vi "C8855-01_InitCall.vi"() -> (0 "ExtT":bool, 1 "Moni":bool, 2 "Measur":u32, 3 "GT":i32, 4 "TrgEdge":u8)   [LabVIEW 2017]
panel:
  out "InitFN":string
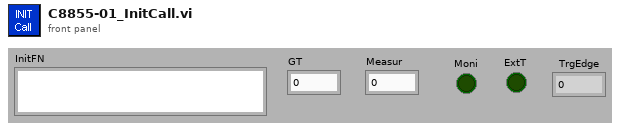
[diagram p1: front panel]
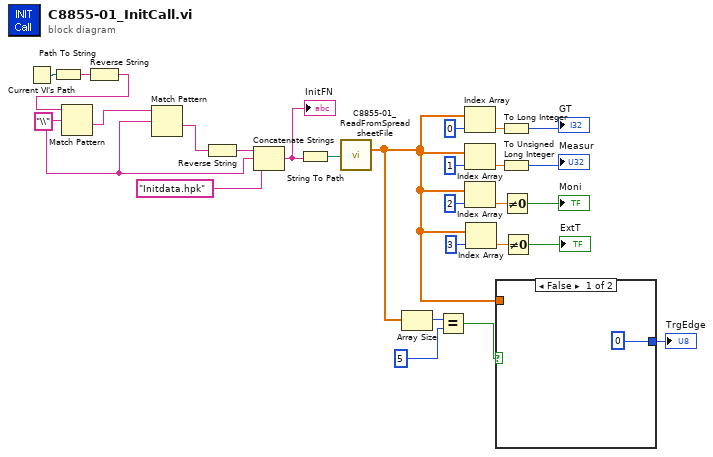
[diagram p0: block diagram]
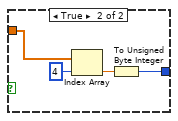
[diagram p2: hidden frame]
diagram:
  w20 = "\\" ("regular expression")
  n1 = Current VI's Path() -> (path=w27:path)
  n2 = Path To String(path=w27) -> (string=w26:string)
  n3 = Reverse String(1:w26) -> (0:w24:string)
  n4 = Match Pattern(string=w24, regular expression=w20) -> (after substring=w21:string)  [unwired: 4 out]
  n5 = Match Pattern(string=w21, regular expression=w20) -> (after substring=w19:string)  [unwired: 4 out]
  n6 = Reverse String(1:w19) -> (0:w25:string)
  n7 = Concatenate Strings(w25, w20, "Initdata.hpk") -> (w22:string)
  "InitFN" <- w22
  n8 = String To Path(string=w22) -> (path=w16:path)
  n9 = call "C8855-01_ReadFromSpreadsheetFile.vi"("file path (dialog if empty)"=w16) -> ("first row"=w2:sgl[])  [unwired: 4 in, 10 out]
  n10 = Array Size(array=w2) -> (size(s)=w5:i32)
  n11 = Equal?(x=w5, y=5) -> (x = y?=w3:bool)
  n12 = Index Array(array=w2, index=0 ("Index")) -> (element=w15:sgl)
  n13 = Index Array(array=w2, index=1 ("Index")) -> (element=w14:sgl)
  n14 = Index Array(array=w2, index=2 ("Index")) -> (element=w12:sgl)
  n15 = Index Array(array=w2, index=3 ("Index")) -> (element=w7:sgl)
  n16 = case shown="FALSE" w3 {
    tunnel: w2 -> [_ w32]
    tunnel: [u8 0 w29] -> w1
    frame False {
    }
    frame True {
      n17 = Index Array(array=w32, index=4 ("指標")) -> (element=w30:sgl)
      n18 = To Unsigned Byte Integer(number=w30) -> (unsigned 8bit integer=w29:u8)
    }
  }
  "TrgEdge" <- w1
  n19 = To Long Integer(number=w15) -> (32bit integer=→"GT":i32)
  n20 = To Unsigned Long Integer(number=w14) -> (unsigned 32bit integer=→"Measur":u32)
  n21 = Not Equal To 0?(x=w12) -> (x != 0?=→"Moni":bool)
  n22 = Not Equal To 0?(x=w7) -> (x != 0?=→"ExtT":bool)
